vi "p2.vi"() -> ()   [LabVIEW 2023, in "d19.lvlib"]
uses:
  d19.lvlib
  Users/Standard/OneDrive - Argenta/Desktop/SubPanel Actors/GUI/GUI/Rule Type.ctl
  <vilib>/regexp/Match Regular Expression.xnode
  AOC/AOC.lvlib
panel:
  in  "Example":string="px{a<2006:qkq,m>2090:A,rfg}\npv{a>1716:R,A}\nlnx{m>1548:A,A}\nrfg{s<537:gd,x>2440:R,A}\nqs{s>3448:A,lnx}\nqkq{x<1416:A,crn}\ncrn{x>2662:A,R}\nin{s<1351:px,qqz}\nqqz{s>2770:qs,m<1801:hdj,R}\ngd{a>3333:R,R}\nhdj{m>838:A,pv}\n\n{x=787,m=2655,a=1222,s=2876}\n{x=1679,m=44,a=2067,s=496}\n{x=2036,m=264,a=79,s=2244}\n{x=2461,m=1339,a=466,s=291}\n{x=2127,m=1623,a=2188,s=1013}"
  in  "Example":bool=TRUE
  out "Answer":u64=978
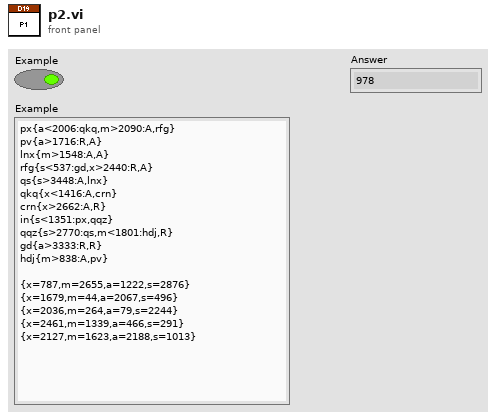
[diagram p1: front panel]
types:
  T1 = cluster{"Rule Type":string, "Index":i32, "Label":string}[]
  T2 = typedef "d19.lvlib/Rule Type.ctl" = enum16{"<", ">", "R", "A", "goto"}
  T3 = map{string, cluster{"Type":T2, "Route":string, "Rating":u8, "Value":i32}[]}
  T4 = cluster{"Type":T2, "whole match":string, "default value 1":u8, i32}
  T5 = cluster{string, "Rule Index":i32, cluster{"First Rating":u64, "Last Rating":u64}[]}
  T6 = cluster{string, "Rule Index":i32, cluster{"First Rating":u64, "Last Rating":u64}[]}[]
  T7 = cluster{"Type":T2, "Route":string, "Rating":u8, "Value":i32}[]
  T8 = cluster{"Type":T2, "Route":string, "Rating":u8, "Value":i32}
  T9 = cluster{"Route":string, i32, cluster{"First Rating":u64, "Last Rating":u64}[]}
  T10 = cluster{string, i32, cluster{"First Rating":u64, "Last Rating":u64}[]}
  T11 = cluster{"Route":string, "Rule Index":i32, cluster{"First Rating":u64, "Last Rating":u64}[]}
  T12 = cluster{"Route":string, "Rule Index":i32, cluster{"First Rating":u64, "Last Rating":u64}[]}[]
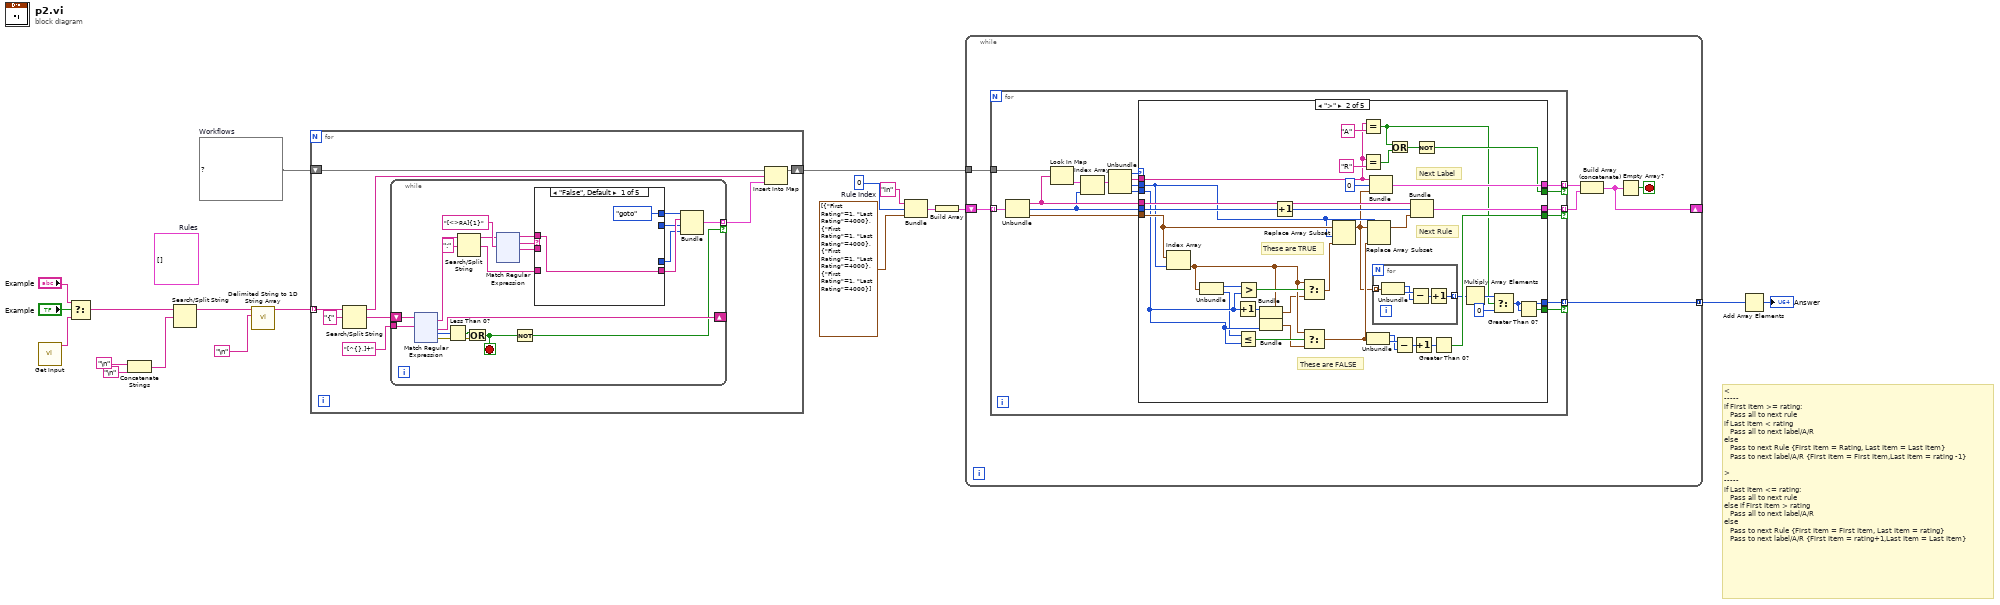
[diagram p0: block diagram]
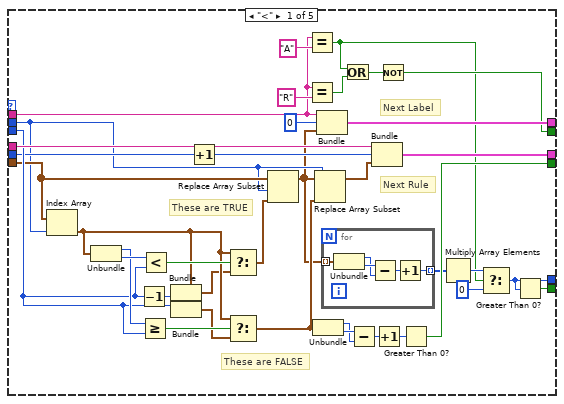
[diagram p2: hidden frame]
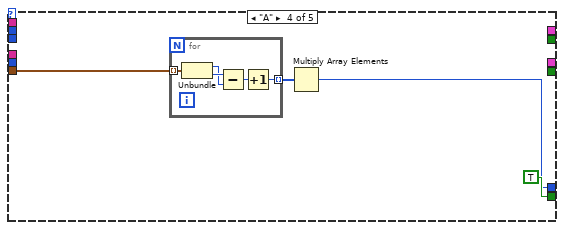
[diagram p4: hidden frame]
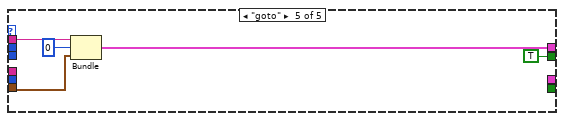
[diagram p5: hidden frame]
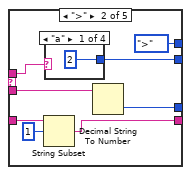
[diagram p6: hidden frame]
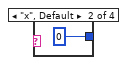
[diagram p7: hidden frame]
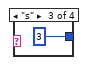
[diagram p8: hidden frame]
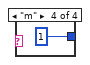
[diagram p9: hidden frame]
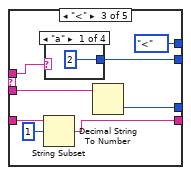
[diagram p10: hidden frame]
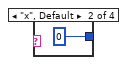
[diagram p11: hidden frame]
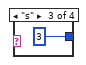
[diagram p12: hidden frame]
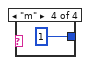
[diagram p13: hidden frame]
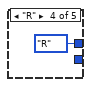
[diagram p14: hidden frame]
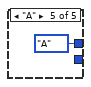
[diagram p15: hidden frame]
diagram:
  w2 = 0  # Rule Index
  (unwired) T1 []  # Rules
  w10 = T3 {}  # Workflows
  # "<\n-----\nif First Item >= rating:\n   Pass all to next rule\nif Last Item < rating\n   Pass all to next label/A/R\nelse\n   Pass to next Rule {First Item = Rating, Last Item = Last Item}\n   Pass to next label/A/R {First Item = First Item,Last Item = rating -1}\n\n>\n-----\nif Last Item <= rating:\n   Pass all to next rule\nelse if First Item > rating\n   Pass all to next label/A/R\nelse\n   Pass to next Rule {First Item = First Item, Last Item = rating}\n   Pass to next label/A/R {First Item = rating+1,Last Item = Last Item}"
  n1 = call "Get Input.vi"() -> ("Input"=w19:string)  [unwired: 11 in]
  n2 = Select(t="Example", s="Example", f=w19) -> (s? t:f=w16:string)
  n3 = Concatenate Strings("\n", "\n") -> (w13:string)
  n4 = Search/Split String(string=w16, search string/char (-)=w13) -> (substring before match=w12:string)  [unwired: 1 in, 2 out]
  n5 = call <vilib>:"Delimited String to 1D String Array.vi"("delimiter"="\n", "delimited string"=w12) -> ("string array"=w11:string[])  [unwired: 9 in]
  n6 = for {
    tunnel: w11 -> [w25] mode=indexing
    shift-right: [w26] -> w8
    shift-left: w10 -> [w27]
    n7 = Search/Split String(string=w25, search string/char (-)="{") -> (substring before match=w23:string, match + rest of string=w22:string)  [unwired: 1 in, 1 out]
    n8 = while {
      shift-right: [w47] -> _
      shift-left: w22 -> [w48]
      tunnel: [w32] -> w20 mode=indexing if=w41
      tunnel: "[^{},]+" -> [w46]
      stop <- w42 stop-if-true
      n9 = xnode "Match Regular Expression"("input string"=w48, "regular expression"=w46) -> ("whole match"=w30:string, "after match"=w47:string, "offset past match"=w45:i32, "error out"=w43:errorcluster)  [unwired: 4 in, 1 out]
      n10 = Less Than 0?(x=w45) -> (x < 0?=w44:bool)
      n11 = Search/Split String(string=w30, search string/char (-)=":") -> (substring before match=w29:string, match + rest of string=w28:string)  [unwired: 1 in, 1 out]
      n12 = Or(x=w44, y=w43) -> (x .or. y?=w42:bool)
      n13 = xnode "Match Regular Expression"("input string"=w29, "regular expression"="[<>RA]{1}") -> ("before match"=w38:string, "whole match"=w39:string, "after match"=w37:string)  [unwired: 4 in, 2 out]
      n14 = Not(x=w42) -> (.not. x?=w41:bool)
      n15 = case shown="\"False\", Default" w39 {
        tunnel: [Rule_Type."goto" ("Type") Rule_Type.">" ("Type") Rule_Type."<" ("Type") Rule_Type."R" ("Type") Rule_Type."A" ("Type")] -> w36
        tunnel: w38 -> [w50 w56 w68 _ _]
        tunnel: w37 -> [_ w54 w66 _ _]
        tunnel: [_ w55 w67 _ _] -> w34
        tunnel: [_ w57 w69 _ _] -> w33
        tunnel: [w50 w52 w64 _ _] -> w35
        tunnel: w28 -> [_ w53 w65 _ _]
        frame "False", Default {
        }
        frame ">" {
          n16 = String Subset(string=w53, offset (0)=1) -> (substring=w52:string)  [unwired: 1 in]
          n17 = case shown="\"a\"" w56 {
            tunnel: [u8 2 ("default value 1") u8 0 ("default value 1") u8 3 ("default value 1") u8 1 ("default value 1")] -> w55
            frame "a" {
            }
            frame "x", Default {
            }
            frame "s" {
            }
            frame "m" {
            }
          }
          n18 = Decimal String To Number(string=w54) -> (number=w57:i32)  [unwired: 2 in, 1 out]
        }
        frame "<" {
          n19 = String Subset(string=w65, offset (0)=1) -> (substring=w64:string)  [unwired: 1 in]
          n20 = case shown="\"a\"" w68 {
            tunnel: [u8 2 ("default value 1") u8 0 ("default value 1") u8 3 ("default value 1") u8 1 ("default value 1")] -> w67
            frame "a" {
            }
            frame "x", Default {
            }
            frame "s" {
            }
            frame "m" {
            }
          }
          n21 = Decimal String To Number(string=w66) -> (number=w69:i32)  [unwired: 2 in, 1 out]
        }
        frame "R" {
        }
        frame "A" {
        }
      }
      n22 = Bundle("Type"=w36, "whole match"=w35, "default value 1"=w34, w33) -> (w32:T4)  [unwired: 1 in]
    }
    n23 = Insert Into Map(map in=w27, key=w23, value=w20) -> (map out=w26:T3)  [unwired: 2 out]
  }
  n24 = Bundle("in", "Rule Index"=w2, cluster{"First Rating":u64, "Last Rating":u64}[] [{"First Rating"=1, "Last Rating"=4000}, {"First Rating"=1, "Last Rating"=4000}, {"First Rating"=1, "Last Rating"=4000}, {"First Rating"=1, "Last Rating"=4000}]) -> (w7:T5)  [unwired: 1 in]
  n25 = Build Array(w7) -> (w5:T6)
  n26 = while {
    tunnel: w8 -> [w317]
    shift-right: [w312] -> _
    shift-left: w5 -> [w316]
    tunnel: [w315] -> w1 mode=concatenating
    stop <- w311 stop-if-true
    n27 = for {
      tunnel: w317 -> [w333]
      tunnel: w316 -> [w318] mode=indexing
      tunnel: [w322] -> w315 mode=indexing if=w321
      tunnel: [w323] -> w313 mode=indexing if=w319
      tunnel: [w324] -> w314 mode=indexing if=w320
      n28 = Unbundle(w318) -> (w326:string, "Rule Index"=w325:i32, w332:cluster{"First Rating":u64, "Last Rating":u64}[])
      n29 = Look In Map(map=w333, key=w326) -> (value=w334:T7)  [unwired: 1 in, 1 out]
      n30 = Index Array(array=w334, index=w325) -> (element=w327:T8)
      n31 = Unbundle(w327) -> ("Type"=w331:T2, "Route"=w330:string, "Rating"=w329:u8, "Value"=w328:i32)
      n32 = case shown="\">\"" w331 {
        tunnel: w332 -> [w344 w392 _ w422 w432]
        tunnel: w330 -> [w360 w406 _ _ w434]
        tunnel: w329 -> [w343 w391 _ _ _]
        tunnel: w328 -> [w358 w386 _ _ _]
        tunnel: [w355 w402 _ _ _] -> w323
        tunnel: w326 -> [w361 w407 _ _ _]
        tunnel: w325 -> [w357 w404 _ _ _]
        tunnel: [w351 w398 _ _ w431] -> w324
        tunnel: [w347 w395 _ w421 _] -> w322
        tunnel: [w348 w396 _ TRUE _] -> w321
        tunnel: [w340 w388 _ _ TRUE] -> w320
        tunnel: [w339 w387 _ _ _] -> w319
        frame "<" {
          # "Next Rule"
          # "Next Label"
          # "These are TRUE"
          # "These are FALSE"
          n33 = Index Array(array=w344, index=w343) -> (element=w364:cluster{"First Rating":u64, "Last Rating":u64})
          n34 = Unbundle(w364) -> ("First Rating"=w366:u64, "Last Rating"=w368:u64)
          n35 = Decrement(x=w358) -> (x-1=w363:i32)
          n36 = Greater Or Equal?(x=w366, y=w358) -> (x >= y?=w369:bool)
          n37 = Less?(x=w368, y=w358) -> (x < y?=w365:bool)
          n38 = Bundle(cluster=w364, "Last Rating"=w363) -> (w362:cluster{"First Rating":u64, "Last Rating":u64})  [unwired: 1 in]
          n39 = Bundle(cluster=w364, "First Rating"=w358) -> (w367:cluster{"First Rating":u64, "Last Rating":u64})  [unwired: 1 in]
          n40 = Increment(x=w357) -> (x+1=w356:i32)
          n41 = Select(t=w364, s=w365, f=w362) -> (s? t:f=w342:cluster{"First Rating":u64, "Last Rating":u64})
          n42 = Select(t=w364, s=w369, f=w367) -> (s? t:f=w346:cluster{"First Rating":u64, "Last Rating":u64})
          n43 = Replace Array Subset(array=w344, new element=w342, index=w343) -> (w338:cluster{"First Rating":u64, "Last Rating":u64}[])
          n44 = Equal?(x=w360, y="A") -> (x = y?=w335:bool)
          n45 = Equal?(x=w360, y="R") -> (x = y?=w350:bool)
          n46 = Unbundle(w346) -> ("First Rating"=w353:u64, "Last Rating"=w354:u64)
          n47 = Replace Array Subset(array=w338, new element=w346, index=w343) -> (w345:cluster{"First Rating":u64, "Last Rating":u64}[])
          n48 = Bundle("Route"=w360, 0, w338) -> (w351:T9)  [unwired: 1 in]
          n49 = for {
            tunnel: [w374] -> w337 mode=indexing
            tunnel: w338 -> [w373] mode=indexing
            n50 = Unbundle(w373) -> ("First Rating"=w376:u64, "Last Rating"=w377:u64)
            n51 = Subtract(x=w377, y=w376) -> (x-y=w375:u64)
            n52 = Increment(x=w375) -> (x+1=w374:u64)
          }
          n53 = Or(x=w335, y=w350) -> (x .or. y?=w372:bool)
          n54 = Subtract(x=w354, y=w353) -> (x-y=w352:u64)
          n55 = Bundle(w361, w356, w345) -> (w355:T10)  [unwired: 1 in]
          n56 = Increment(x=w352) -> (x+1=w341:u64)
          n57 = Not(x=w372) -> (.not. x?=w340:bool)
          n58 = Greater Than 0?(x=w341) -> (x > 0?=w339:bool)
          n59 = Multiply Array Elements(1:w337) -> (0:w336:u64)
          n60 = Select(t=w336, s=w335, f=u64 0 ("t")) -> (s? t:f=w347:u64)
          n61 = Greater Than 0?(x=w347) -> (x > 0?=w348:bool)
        }
        frame ">" {
          # "Next Rule"
          # "Next Label"
          # "These are TRUE"
          # "These are FALSE"
          n62 = Index Array(array=w392, index=w391) -> (element=w409:cluster{"First Rating":u64, "Last Rating":u64})
          n63 = Unbundle(w409) -> ("First Rating"=w383:u64, "Last Rating"=w384:u64)
          n64 = Increment(x=w386) -> (x+1=w385:i32)
          n65 = Less Or Equal?(x=w384, y=w386) -> (x <= y?=w412:bool)
          n66 = Greater?(x=w383, y=w386) -> (0:w410:bool)
          n67 = Bundle(cluster=w409, "First Rating"=w385) -> (w408:cluster{"First Rating":u64, "Last Rating":u64})  [unwired: 1 in]
          n68 = Bundle(cluster=w409, "Last Rating"=w386) -> (w411:cluster{"First Rating":u64, "Last Rating":u64})  [unwired: 1 in]
          n69 = Increment(x=w404) -> (x+1=w403:i32)
          n70 = Select(t=w409, s=w410, f=w408) -> (s? t:f=w390:cluster{"First Rating":u64, "Last Rating":u64})
          n71 = Select(t=w409, s=w412, f=w411) -> (s? t:f=w394:cluster{"First Rating":u64, "Last Rating":u64})
          n72 = Replace Array Subset(array=w392, new element=w390, index=w391) -> (w382:cluster{"First Rating":u64, "Last Rating":u64}[])
          n73 = Equal?(x=w406, y="A") -> (x = y?=w379:bool)
          n74 = Equal?(x=w406, y="R") -> (x = y?=w378:bool)
          n75 = Unbundle(w394) -> ("First Rating"=w400:u64, "Last Rating"=w401:u64)
          n76 = Replace Array Subset(array=w382, new element=w394, index=w391) -> (w393:cluster{"First Rating":u64, "Last Rating":u64}[])
          n77 = Bundle("Route"=w406, 0, w382) -> (w398:T9)  [unwired: 1 in]
          n78 = for {
            tunnel: [w417] -> w381 mode=indexing
            tunnel: w382 -> [w416] mode=indexing
            n79 = Unbundle(w416) -> ("First Rating"=w419:u64, "Last Rating"=w420:u64)
            n80 = Subtract(x=w420, y=w419) -> (x-y=w418:u64)
            n81 = Increment(x=w418) -> (x+1=w417:u64)
          }
          n82 = Or(x=w379, y=w378) -> (x .or. y?=w415:bool)
          n83 = Subtract(x=w401, y=w400) -> (x-y=w399:u64)
          n84 = Bundle(w407, w403, w393) -> (w402:T10)  [unwired: 1 in]
          n85 = Increment(x=w399) -> (x+1=w389:u64)
          n86 = Not(x=w415) -> (.not. x?=w388:bool)
          n87 = Greater Than 0?(x=w389) -> (x > 0?=w387:bool)
          n88 = Multiply Array Elements(1:w381) -> (0:w380:u64)
          n89 = Select(t=w380, s=w379, f=u16 0 ("t")) -> (s? t:f=w395:u64)
          n90 = Greater Than 0?(x=w395) -> (x > 0?=w396:bool)
        }
        frame "R" {
        }
        frame "A" {
          n91 = for {
            tunnel: [w426] -> w423 mode=indexing
            tunnel: w422 -> [w425] mode=indexing
            n92 = Unbundle(w425) -> ("First Rating"=w428:u64, "Last Rating"=w429:u64)
            n93 = Subtract(x=w429, y=w428) -> (x-y=w427:u64)
            n94 = Increment(x=w427) -> (x+1=w426:u64)
          }
          n95 = Multiply Array Elements(1:w423) -> (0:w421:u64)
        }
        frame "goto" {
          n96 = Bundle("Route"=w434, "Rule Index"=0, w432) -> (w431:T11)  [unwired: 1 in]
        }
      }
    }
    n97 = Build Array (concatenate)(w314, w313) -> (w312:T12)
    n98 = Empty Array?(array=w312) -> (empty?=w311:bool)
  }
  n99 = Add Array Elements(numeric array=w1) -> (sum=→"Answer":u64)
